vi "parse_parameters.vi"(8 "error in (no error)":errorcluster, 11 "Fixed Parameters":string[][](table)=[["inital period (ms)", "i", "500", "4000", "1"], ["Overall period (ms)", "t", "6000", "8000", "1"], ["rabi time (ms)", "r", "1", "1", "1"], ["repump delay", "q", "20", "20", "1"], ["push beam", "p", "0", "0", "1"], ["optical pumping", "a", "20", "20", "1"], ["", "b", "1", "1", "1"], ["", "c", "1", "1", "1"]] caption="(variables that do not iterate)") -> (0 "error out":errorcluster, 2 "paramter values":dbl[](array[numeric]), 3 "Parameter names":string[](array[string]))   [LabVIEW 2013]
doc: "1. Saves off the first column of data as \"plot axis labels\" in \"Processed Data.txt\"\n2. Go through all the possible iterations of the variables, and output a 2D array of those iterations.\n3. Save the data ordering into \"Data Order Log.txt\""
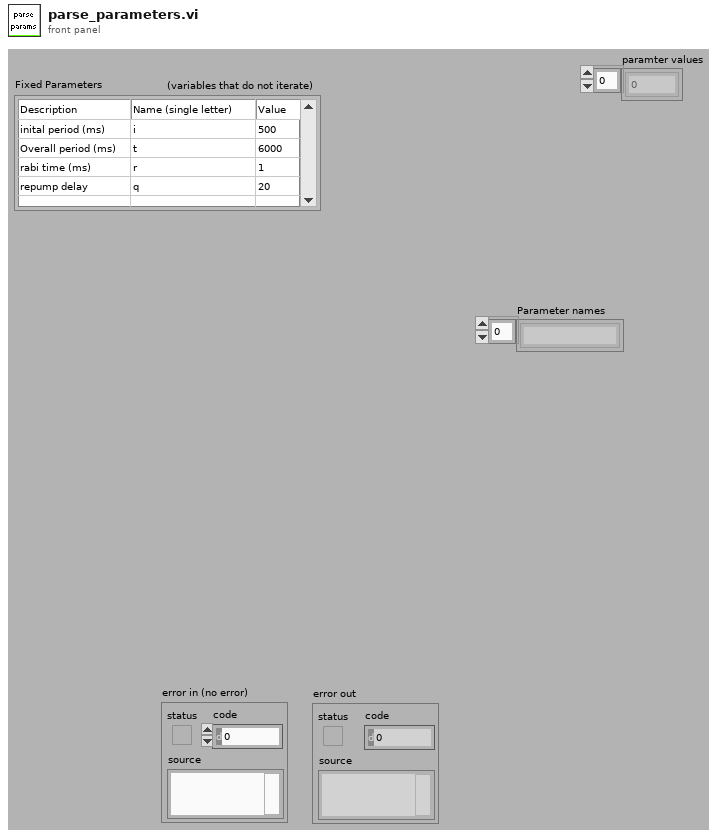
[diagram p1: front panel]
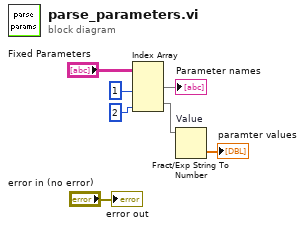
[diagram p0: block diagram]
diagram:
  n1 = Index Array(array="Fixed Parameters", index (col) #1=1 ("disabled index (col)"), index (col) #2=2 ("index (col)")) -> (element #1=→"Parameter names":string[], element #2=w3:string[])  [unwired: 2 in]
  n2 = Fract/Exp String To Number "Value"(string=w3) -> (number=→"paramter values":dbl[])  [unwired: 3 in, 1 out]
  "error out" <- "error in (no error)"
